vi "Autonomous Independent.vi"() -> ()   [LabVIEW 2011]
doc: "This VI is called when autonomous begins, and will automatically be terminated when autonomous ends. You can carry out timed or sensor driven robot movement independently without needing to return to the caller."
uses:
  Robot Global Data.vi
panel:
  in  "Recording Auton":bool
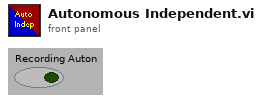
[diagram p1: front panel]
types:
  T1 = typedef "WPI_MotorControlDeviceRef.ctl" = cluster{"DeviceStatus":errorcluster, "Type":enum16{"PWM", "CAN"}, "PWM":cluster{"Digital Module":T2, "PWM Channel":T3, "DeadBand":T4}, "CAN":cluster{"Device Number":u8, "Control Mode":T5, "Semaphore":T6, "Max Vout":dbl}, "Invert":bool, "TransformRef":T7, "InvTransformRef":T7}
  T2 = typedef "FPGA_TypedefDigitalModule.ctl" = enum16{"Digital Module 1", "Digital Module 2"}
  T3 = typedef "FPGA_DIOPWMChannel.ctl" = enum8{"PWM 1", "PWM 2", "PWM 3", "PWM 4", "PWM 5", "PWM 6", "PWM 7", "PWM 8", "PWM 9", "PWM 10", "Invalid"}
  T4 = typedef "WPI_PWMDeadband.ctl" = cluster{"Name":string, "maxPositivePwm":i32, "minPositivePwm":i32, "centerPwm":i32, "maxNegativePwm":i32, "minNegativePwm":i32, "angularRange":u16}
  T5 = typedef "WPI_CANJaguar_ControlMode.ctl" = enum8{"Percent VBus", "Current", "Speed", "Position", "Voltage"}
  T6 = typedef "Semaphore RefNum" = refnum<k1>
  T7 = typedef "WPI_PWMTransform_ConPane.ctl" = refnum<vi>
  T8 = typedef "WPI_ServoDeviceRef.ctl" = cluster{"DeviceStatus":errorcluster, "Digital Module":T2, "PWM Channel":T3, "DeadBand":T4}
  T9 = typedef "WPI_EncoderDevRef.ctl" = cluster{"DevStatus":errorcluster, "EncoderIndex":T10, "CounterIndex":T11, "DistancePerCount":dbl, "Decoding Type":T12}
  T10 = typedef "FPGA_EncoderIdx.ctl" = enum8{"Enc 0", "Enc 1", "Enc 2", "Enc 3", "Invalid"}
  T11 = typedef "FPGA_CounterCtrSystemIndex.ctl" = enum8{"Ctr 0", "Ctr 1", "Ctr 2", "Ctr 3", "Ctr 4", "Ctr 5", "Ctr 6", "Ctr 7", "Invalid"}
  T12 = typedef "WPI_EncoderType.ctl" = enum16{"1x", "2x", "4x"}
  T13 = typedef "WPI_GyroDevRef.ctl" = cluster{"DevStatus":errorcluster, "Analog Module":T14, "Analog Channel":T15, "Offset":dbl, "Gain (VoltsPerDegree/Second)":dbl}
  T14 = typedef "FPGA_TypedefAnalogModule.ctl" = enum16{"Analog Module 1", "Analog Module 2"}
  T15 = typedef "FPGA_AIChannel.ctl" = enum8{"AI 1", "AI 2", "AI 3", "AI 4", "AI 5", "AI 6", "AI 7", "AI 8", "Invalid"}
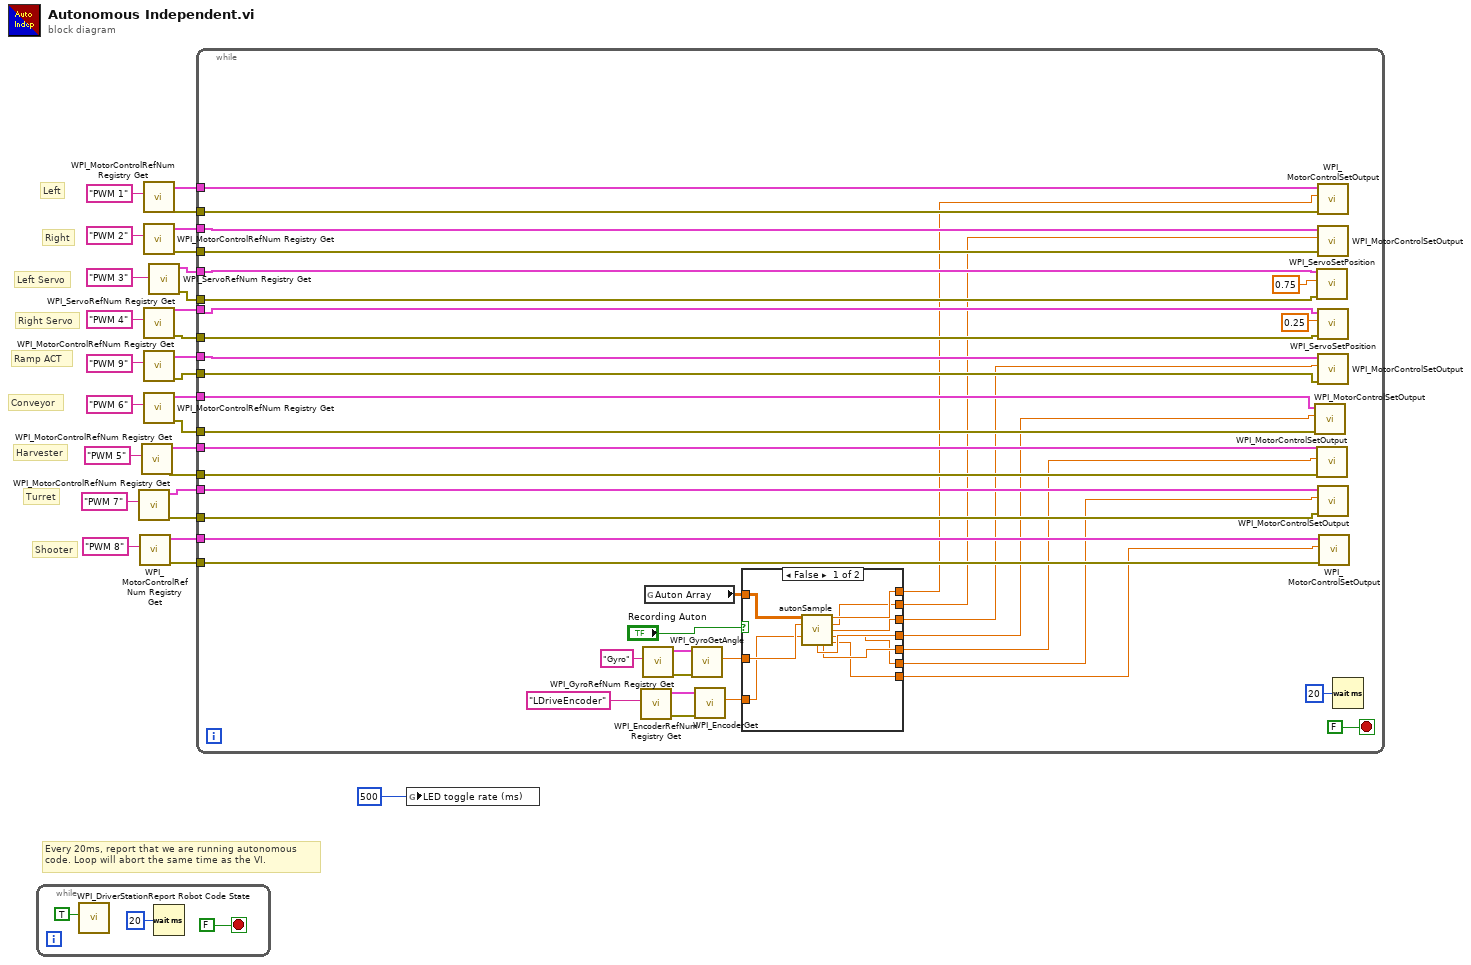
[diagram p0: block diagram]
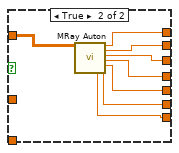
[diagram p2: hidden frame]
diagram:
  # "Shooter"
  # "Turret"
  # "Conveyor"
  # "Harvester"
  # "Ramp ACT"
  # "Right Servo"
  # "Left Servo"
  # "Right"
  # "Left"
  # "Every 20ms, report that we are running autonomous\ncode. Loop will abort the same time as the VI."
  n1 = while {
    stop <- FALSE stop-if-true
    n2 = call <vilib>:"WPI_DriverStationReport Robot Code State.vi"("Autonomous"=TRUE) -> ()  [unwired: 10 in, 1 out]
    n3 = Wait (ms)(milliseconds to wait=u32 20) -> ()  [unwired: 1 out]
  }
  n4 = call <vilib>:"WPI_MotorControlRefNum Registry Get.vi"("refnum name"="PWM 7") -> ("error out"=w8:errorcluster, "MotorControlDevRef"=w9:T1)  [unwired: 9 in]
  n5 = call <vilib>:"WPI_MotorControlRefNum Registry Get.vi"("refnum name"="PWM 8") -> ("error out"=w6:errorcluster, "MotorControlDevRef"=w7:T1)  [unwired: 9 in]
  n6 = call <vilib>:"WPI_MotorControlRefNum Registry Get.vi"("refnum name"="PWM 5") -> ("error out"=w10:errorcluster, "MotorControlDevRef"=w11:T1)  [unwired: 9 in]
  n7 = call <vilib>:"WPI_MotorControlRefNum Registry Get.vi"("refnum name"="PWM 1") -> ("error out"=w1:errorcluster, "MotorControlDevRef"=w23:T1)  [unwired: 9 in]
  n8 = call <vilib>:"WPI_MotorControlRefNum Registry Get.vi"("refnum name"="PWM 2") -> ("error out"=w2:errorcluster, "MotorControlDevRef"=w22:T1)  [unwired: 9 in]
  n9 = call <vilib>:"WPI_ServoRefNum Registry Get.vi"("refnum name"="PWM 4") -> ("error out"=w4:errorcluster, "ServoDeviceRef"=w21:T8)  [unwired: 9 in]
  n10 = call <vilib>:"WPI_MotorControlRefNum Registry Get.vi"("refnum name"="PWM 9") -> ("error out"=w5:errorcluster, "MotorControlDevRef"=w20:T1)  [unwired: 9 in]
  n11 = call <vilib>:"WPI_MotorControlRefNum Registry Get.vi"("refnum name"="PWM 6") -> ("error out"=w15:errorcluster, "MotorControlDevRef"=w16:T1)  [unwired: 9 in]
  n12 = call <vilib>:"WPI_ServoRefNum Registry Get.vi"("refnum name"="PWM 3") -> ("error out"=w3:errorcluster, "ServoDeviceRef"=w18:T8)  [unwired: 9 in]
  n13 = while {
    tunnel: w23 -> [w68]
    tunnel: w22 -> [w67]
    tunnel: w18 -> [w62]
    tunnel: w21 -> [w63]
    tunnel: w20 -> [w66]
    tunnel: w16 -> [w61]
    tunnel: w15 -> [w60]
    tunnel: w11 -> [w59]
    tunnel: w10 -> [w58]
    tunnel: w9 -> [w57]
    tunnel: w8 -> [w56]
    tunnel: w7 -> [w55]
    tunnel: w6 -> [w54]
    tunnel: w5 -> [w53]
    tunnel: w4 -> [w52]
    tunnel: w3 -> [w51]
    tunnel: w2 -> [w50]
    tunnel: w1 -> [w49]
    stop <- FALSE stop-if-true
    n14 = call <vilib>:"WPI_EncoderRefNum Registry Get.vi"("refnum name"="LDriveEncoder") -> ("error out"=w38:errorcluster, "EncoderDevRef"=w39:T9)  [unwired: 9 in]
    n15 = call <vilib>:"WPI_GyroRefNum Registry Get.vi"("refnum name"="Gyro") -> ("error out"=w36:errorcluster, "GyroDevRef"=w37:T13)  [unwired: 9 in]
    n16 = global read "Robot Global Data.vi" "Auton Array"() -> (w48:dbl[][])
    n17 = call <vilib>:"WPI_GyroGetAngle.vi"("error in (no error)"=w36, "GyroDevRef"=w37) -> ("Angle"=w33:dbl)  [unwired: 6 in, 3 out]
    n18 = call <vilib>:"WPI_EncoderGet.vi"("error in (no error)"=w38, "EncoderDevRef"=w39) -> ("Distance"=w32:dbl)  [unwired: 4 in, 5 out]
    n19 = case shown="False" "Recording Auton" {
      tunnel: w48 -> [w73 w88]
      tunnel: [w80 w87] -> w47
      tunnel: [w79 w86] -> w46
      tunnel: [w78 w85] -> w45
      tunnel: [w77 w84] -> w44
      tunnel: [w76 w83] -> w43
      tunnel: [w75 w82] -> w42
      tunnel: [w74 w81] -> w41
      tunnel: w33 -> [w72 _]
      tunnel: w32 -> [w71 _]
      frame False {
        n20 = call "autonSample.vi"("Auton Array"=w73, "MeasuredHeading"=w72, "EncoderDistance"=w71) -> ("Left Drive"=w80:dbl, "Right Drive"=w79:dbl, "Ramp ACT motor"=w78:dbl, "Turret Rotation"=w75:dbl, "Conveyor"=w77:dbl, "Harvester"=w76:dbl, "Shooter motor output"=w74:dbl)  [unwired: 6 in]
      }
      frame True {
        n21 = call "MRay Auton.vi"("Auton Array"=w88) -> ("Shooter"=w81:dbl, "Left Drive"=w87:dbl, "Right Drive"=w86:dbl, "Ramp ACT motor"=w85:dbl, "Conveyor"=w84:dbl, "Harvester"=w83:dbl, "Turret Rotation"=w82:dbl)  [unwired: 12 in]
      }
    }
    n22 = call <vilib>:"WPI_MotorControlSetOutput.vi"("error in (no error)"=w60, "Output"=w44, "MotorControlDevRef"=w61) -> ()  [unwired: 7 in, 2 out]
    n23 = call <vilib>:"WPI_ServoSetPosition.vi"("error in (no error)"=w51, "Position"=0.75 ("Output"), "ServoDeviceRef"=w62) -> ()  [unwired: 7 in, 2 out]
    n24 = call <vilib>:"WPI_MotorControlSetOutput.vi"("error in (no error)"=w58, "Output"=w43, "MotorControlDevRef"=w59) -> ()  [unwired: 7 in, 2 out]
    n25 = call <vilib>:"WPI_MotorControlSetOutput.vi"("error in (no error)"=w49, "Output"=w47, "MotorControlDevRef"=w68) -> ()  [unwired: 7 in, 2 out]
    n26 = call <vilib>:"WPI_MotorControlSetOutput.vi"("error in (no error)"=w50, "Output"=w46, "MotorControlDevRef"=w67) -> ()  [unwired: 7 in, 2 out]
    n27 = call <vilib>:"WPI_ServoSetPosition.vi"("error in (no error)"=w52, "Position"=0.25 ("Output"), "ServoDeviceRef"=w63) -> ()  [unwired: 7 in, 2 out]
    n28 = call <vilib>:"WPI_MotorControlSetOutput.vi"("error in (no error)"=w53, "Output"=w45, "MotorControlDevRef"=w66) -> ()  [unwired: 7 in, 2 out]
    n29 = call <vilib>:"WPI_MotorControlSetOutput.vi"("error in (no error)"=w56, "Output"=w42, "MotorControlDevRef"=w57) -> ()  [unwired: 7 in, 2 out]
    n30 = call <vilib>:"WPI_MotorControlSetOutput.vi"("error in (no error)"=w54, "Output"=w41, "MotorControlDevRef"=w55) -> ()  [unwired: 7 in, 2 out]
    n31 = Wait (ms)(milliseconds to wait=u32 20) -> ()  [unwired: 1 out]
  }
  n32 = global write "Robot Global Data.vi" "LED toggle rate (ms)"(u32 500 ("LED ms toggle rate")) -> ()
